vi "send_trigger.vi"(8 "error in (no error)":errorcluster, 10 "message":T1, 11 "GenericDAQ in":refnum<class "GenericDAQ.lvclass">) -> (0 "error out":errorcluster, 3 "GenericDAQ out":refnum<class "GenericDAQ.lvclass">)   [LabVIEW 2010, in "GenericDAQ.lvclass"]
uses:
  GenericDAQ.lvclass
  trigger_enum.ctl
  common/classes/GenericToplevelComponent/GenericToplevelComponent/trigger_type_enum.ctl
  common/classes/ErrorController/ErrorController/class_data.vi
  common/classes/ErrorController/ErrorController/ErrorController.lvclass
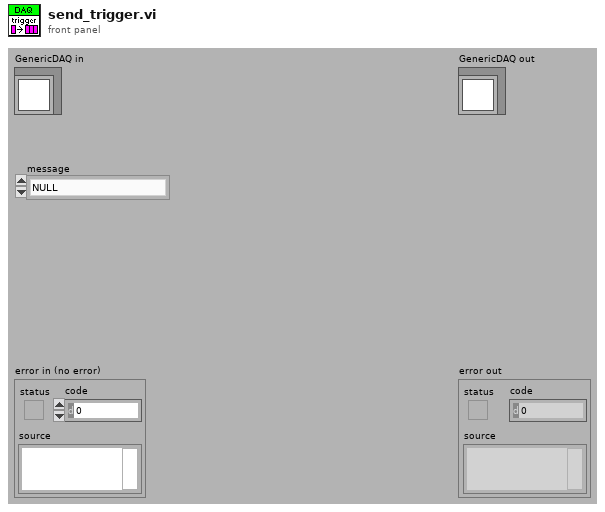
[diagram p1: front panel]
types:
  T1 = typedef "GenericDAQ.lvclass/trigger_enum.ctl" = enum16{"NULL", "read"}
  T2 = typedef "trigger_type_enum.ctl" = enum8{"external", "internal", "common"}
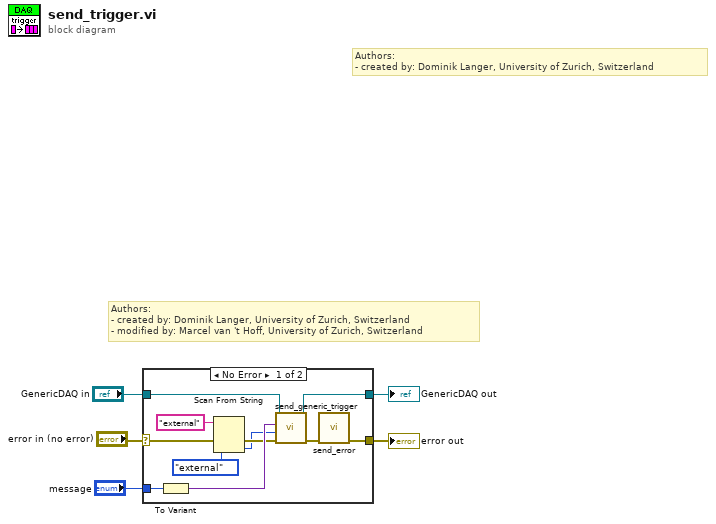
[diagram p0: block diagram]
diagram:
  # "Authors: \n- created by: Dominik Langer, University of Zurich, Switzerland\n- modified by: Marcel van 't Hoff, University of Zurich, Switzerland"
  # "Authors: \n- created by: Dominik Langer, University of Zurich, Switzerland"
  n1 = case shown="No Error" "error in (no error)" {
    selector: "error in (no error)" -> [w10 w18]
    tunnel: [w11 w18] -> w3
    tunnel: "message" -> [w16 _]
    tunnel: "GenericDAQ in" -> [w15 w17]
    tunnel: [w14 w17] -> w1
    frame No Error {
      n2 = To Variant(anything=w16) -> (Variant=w13:variant)
      n3 = Scan From String(input string="external", error in=w10, default 1=trigger_type_enum."external" ("trigger type")) -> (error out=w9:errorcluster, output 1=w6:T2)  [unwired: 2 in, 2 out]
      n4 = call-dynamic "send_generic_trigger.vi"("error in (no error)"=w9, "trigger type"=w6, "trigger variant"=w13, "GenericToplevelComponent in"=w15) -> ("error out"=w12:errorcluster, "GenericToplevelComponent out"=w14:refnum<class "GenericDAQ.lvclass">)  [unwired: 4 in, 2 out]
      n5 = call "send_error.vi"("error in (no error)"=w12) -> ("error out"=w11:errorcluster)  [unwired: 10 in]
    }
    frame Error {
    }
  }
  "error out" <- w3
  "GenericDAQ out" <- w1
